vi "Rectangle Comparison.vi"(6 "Line Border":cluster{"Top":dbl, "Bottom":dbl}={"Top"=6.0, "Bottom"=1.0}, 9 "Second":dbl[](array[numeric]), 11 "First":dbl[](array[numeric])) -> (0 "Rect":T1, 1 "Line":T1, 3 "Scores":T2)   [LabVIEW 2016]
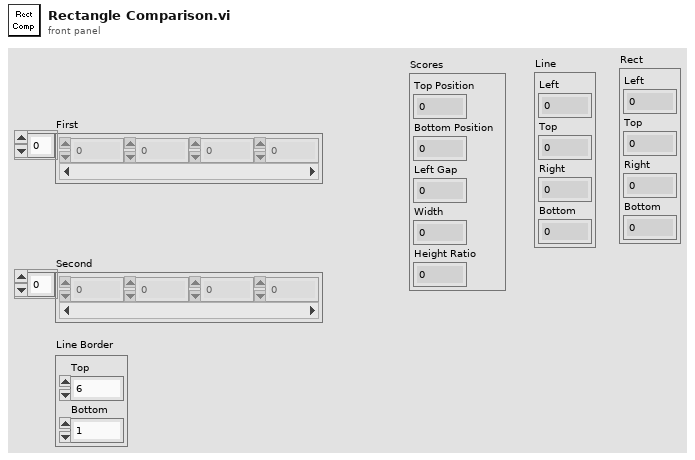
[diagram p1: front panel]
types:
  T1 = cluster{"Left":dbl, "Top":dbl, "Right":dbl, "Bottom":dbl}
  T2 = cluster{"Top Position":dbl, "Bottom Position":dbl, "Left Gap":dbl, "Width":dbl, "Height Ratio":dbl}
  T3 = cluster{"[0]":dbl, "[1]":dbl, "[2]":dbl, "[3]":dbl}
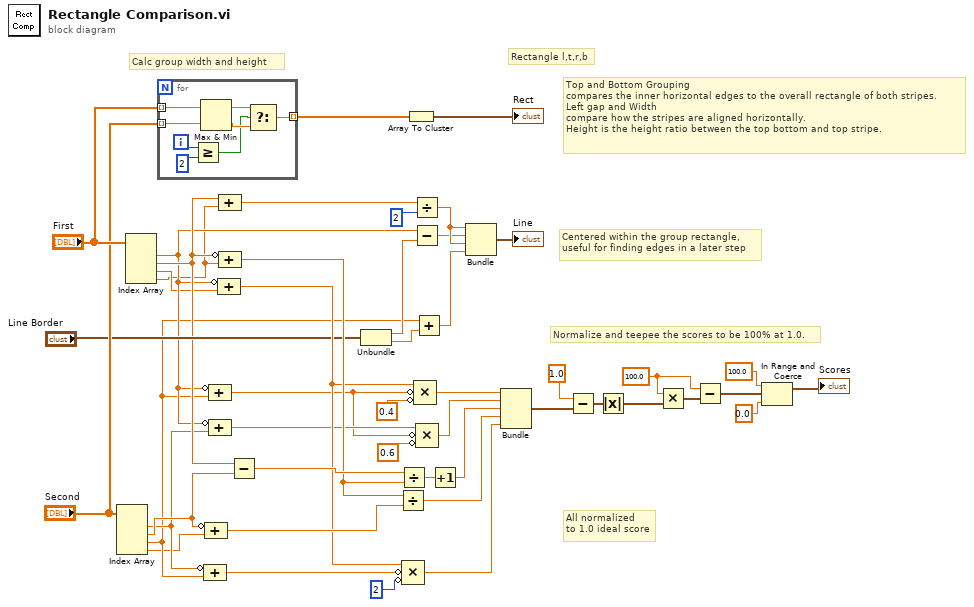
[diagram p0: block diagram]
diagram:
  w25 = 100.0 ("x/y")
  # "Centered within the group rectangle,\nuseful for finding edges in a later step"
  # "All normalized\nto 1.0 ideal score"
  # "Normalize and teepee the scores to be 100% at 1.0."
  # "Top and Bottom Grouping\ncompares the inner horizontal edges to the overall rectangle of both stripes.\nLeft gap and Width\ncompare how the stripes are aligned horizontally.\nHeight is the height ratio between the top bottom and top stripe."
  # "Calc group width and height"
  # "Rectangle l,t,r,b"
  n1 = Index Array(array="Second") -> (element #1=w3:dbl, element #2=w4:dbl, element #3=w2:dbl, element #4=w1:dbl)  [unwired: 4 in]
  n2 = Index Array(array="First") -> (element #1=w7:dbl, element #2=w8:dbl, element #3=w6:dbl, element #4=w5:dbl)  [unwired: 4 in]
  n3 = for {
    tunnel: "First" -> [w55] mode=indexing
    tunnel: "Second" -> [w54] mode=indexing
    tunnel: [w48] -> w32 mode=indexing
    i -> [w52]
    n4 = Greater Or Equal?(x=w52, y=2) -> (x >= y?=w49:bool)
    n5 = Max & Min(x=w55, y=w54) -> (max(x,y)=w51:dbl, min(x,y)=w50:dbl)
    n6 = Select(t=w51, s=w49, f=w50) -> (s? t:f=w48:dbl)
  }
  n7 = Compound Arithmetic op=ADD(invert w3, w2) -> (w46:dbl)
  n8 = Compound Arithmetic op=ADD(invert w4, w1) -> (w47:dbl)
  n9 = Compound Arithmetic op=ADD(invert w7, w2) -> (w15:dbl)
  n10 = Compound Arithmetic op=ADD(invert w7, w3) -> (w16:dbl)
  n11 = Compound Arithmetic op=ADD(invert w7, w6) -> (w17:dbl)
  n12 = Compound Arithmetic op=ADD(w8, w5) -> (w39:dbl)
  n13 = Compound Arithmetic op=ADD(invert w8, w5) -> (w44:dbl)
  n14 = Subtract(x=w8, y=w4) -> (x-y=w45:dbl)
  n15 = Unbundle("Line Border") -> ("Top"=w9:dbl, "Bottom"=w10:dbl)
  n16 = Divide(x=w44, y=w47) -> (x/y=w42:dbl)
  n17 = Divide(x=w45, y=w44) -> (x/y=w40:dbl)
  n18 = Compound Arithmetic op=MULTIPLY(w17, invert w46, invert 2) -> (w41:dbl)
  n19 = Array To Cluster(array=w32) -> (cluster=→"Rect":T3)
  n20 = Divide(x=w39, y=2) -> (x/y=w38:dbl)
  n21 = Subtract(x=w7, y=w9) -> (x-y=w36:dbl)
  n22 = Add(x=w2, y=w10) -> (x+y=w30:dbl)
  n23 = Compound Arithmetic op=MULTIPLY(w17, invert w15, invert 0.4 ("y")) -> (w43:dbl)
  n24 = Compound Arithmetic op=MULTIPLY(w16, invert w15, invert 0.6 ("y")) -> (w14:dbl)
  n25 = Increment(x=w40) -> (x+1=w29:dbl)
  n26 = Bundle(w38, w36, w38, w30) -> (→"Line":cluster{dbl, dbl, dbl, dbl})  [unwired: 1 in]
  n27 = Bundle(w43, w14, w29, w42, w41) -> (w19:cluster{dbl, dbl, dbl, dbl, dbl})  [unwired: 1 in]
  n28 = Subtract(x=1.0 ("y"), y=w19) -> (x-y=w23:cluster{dbl, dbl, dbl, dbl, dbl})
  n29 = Absolute Value(x=w23) -> (abs(x)=w26:cluster{dbl, dbl, dbl, dbl, dbl})
  n30 = Multiply(x=w25, y=w26) -> (x*y=w27:cluster{dbl, dbl, dbl, dbl, dbl})
  n31 = Subtract(x=w25, y=w27) -> (x-y=w22:cluster{dbl, dbl, dbl, dbl, dbl})
  n32 = In Range and Coerce(upper limit=100.0, x=w22, lower limit=0.0) -> (coerced(x)=→"Scores":cluster{dbl, dbl, dbl, dbl, dbl})  [unwired: 1 out]
